vi "Initialize Routing Channel Page.vi"(8 "error in (no error)":errorcluster, 9 "Channel Editor State":T1={"Modules and Connections"=[{" Module Path"="", "Short Module Path"="", "Product Name"="", "Possible Connections"=[], "Missing"=FALSE}, {" Module Path"="", "Short Module Path"="", "Product Name"="", "Possible Connections"=[], "Missing"=FALSE}], "Alias Mappings UI"=[], "Mappings by Module UI"=[]}, 10 "Routing Channel Page Controls":T8, 11 "Routing Channel Ref in":T7 format="%.0x") -> (0 "error out":errorcluster, 3 "Routing Channel Ref out":T7 format="%.0x")   [LabVIEW 2020, in "Routing and Faulting System Explorer.lvlib"]
uses:
  Routing and Faulting System Explorer.lvlib
  <vilib>/NI VeriStand/Custom Device API/Custom Device Item Ref.ctl
  Routing Channel Page Controls.ctl
  Channel Editor State.ctl
  Possible Connections.ctl
  Shared/Routing and Faulting Hardware API/Types/Possible Connections for Endpoint.ctl
  Shared/Alias Mapping.ctl
  Shared/Alias Endpoint.ctl
  Alias Map by Module.ctl
  <vilib>/NI VeriStand/Custom Device API/Custom Device API.lvlib
  Shared/Routing and Faulting Shared.lvlib
  Shared/Routing and Faulting Hardware API/Routing and Faulting Hardware API.lvlib
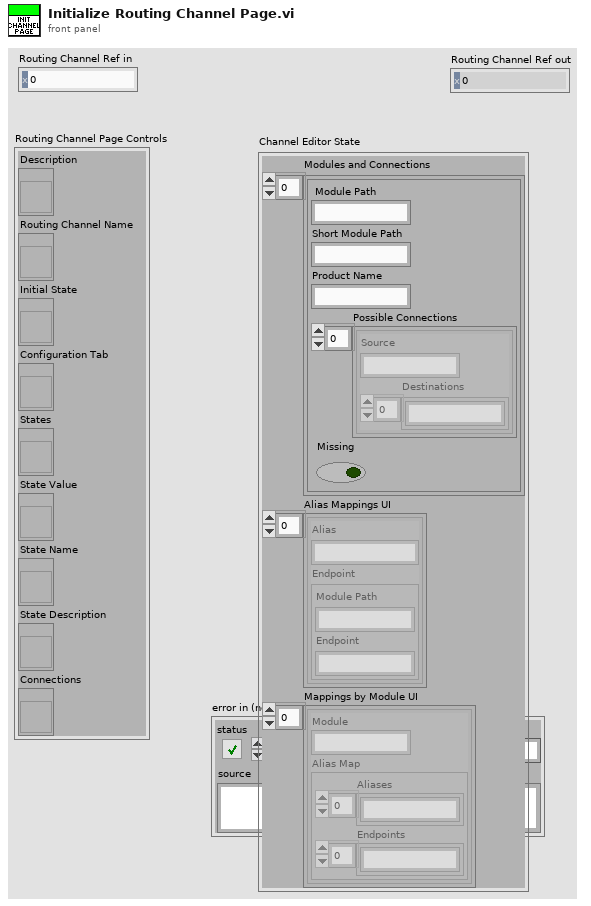
[diagram p1: front panel]
types:
  T1 = typedef "Routing and Faulting System Explorer.lvlib/Channel Editor State.ctl" = cluster{"Modules and Connections":T2[], "Alias Mappings UI":T4[], "Mappings by Module UI":T6[]}
  T2 = typedef "Routing and Faulting System Explorer.lvlib/Possible Connections.ctl" = cluster{" Module Path":string, "Short Module Path":string, "Product Name":string, "Possible Connections":T3[], "Missing":bool}
  T3 = typedef "Routing and Faulting Hardware API.lvlib/Possible Connections for Endpoint.ctl" = cluster{"Source":string, "Destinations":string[]}
  T4 = typedef "Routing and Faulting Shared.lvlib/Alias Mapping.ctl" = cluster{"Alias":string, "Endpoint":T5}
  T5 = typedef "Routing and Faulting Shared.lvlib/Alias Endpoint.ctl" = cluster{"Module Path":string, "Endpoint":string}
  T6 = typedef "Routing and Faulting System Explorer.lvlib/Alias Map by Module.ctl" = cluster{"Module":string, "Alias Map":cluster{"Aliases":string[], "Endpoints":string[]}}
  T7 = typedef "Custom Device API.lvlib/Custom Device Item Ref.ctl" = u64
  T8 = typedef "Routing and Faulting System Explorer.lvlib/Routing Channel Page Controls.ctl" = cluster{"Description":refnum<vi>, "Routing Channel Name":refnum<vi>, "Initial State":refnum<vi>, "Configuration Tab":refnum<vi>, "States":refnum<vi>, "State Value":refnum<vi>, "State Name":refnum<vi>, "State Description":refnum<vi>, "Connections":refnum<vi>}
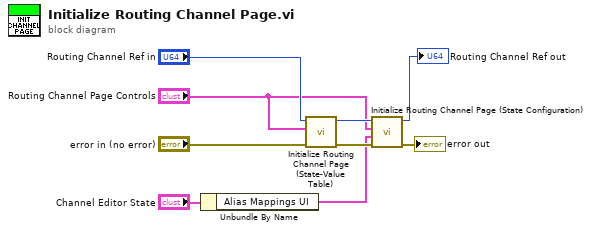
[diagram p0: block diagram]
diagram:
  n1 = Unbundle By Name("Channel Editor State") -> ("Alias Mappings UI"=w1:T4[])
  n2 = call "Initialize Routing Channel Page (State-Value Table).vi"("error in (no error)"="error in (no error)", "Routing Channel Page Controls"="Routing Channel Page Controls", "Routing Channel Ref in"="Routing Channel Ref in") -> ("error out"=w8:errorcluster, "Routing Channel Ref out"=w6:T7)  [unwired: 7 in]
  n3 = call "Initialize Routing Channel Page (State Configuration).vi"("error in (no error)"=w8, "Alias Mappings"=w1, "Routing Channel Page Controls"="Routing Channel Page Controls", "Routing Channel Ref in"=w6) -> ("error out"=→"error out":errorcluster, "Routing Channel Ref out"=→"Routing Channel Ref out":T7)  [unwired: 6 in]
